vi "6（接收方）.vi"() -> ()   [LabVIEW 2017]
panel:
  in  "停止":bool
  out "波形图表":dbl(graph)
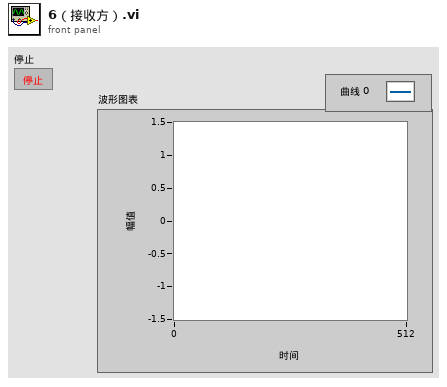
[diagram p1: front panel]
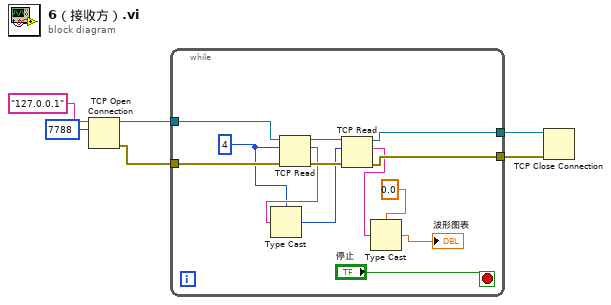
[diagram p0: block diagram]
diagram:
  n1 = TCP Open Connection(address="127.0.0.1" ("地址"), remote port or service name=u16 7788 ("远程端口或服务名称")) -> (connection ID=w6:refnum<k5>, error out=w5:errorcluster)  [unwired: 3 in]
  n2 = while {
    tunnel: w6 -> [w19]
    tunnel: w5 -> [w18]
    tunnel: [w12] -> w4
    tunnel: [w11] -> w3
    stop <- "停止" stop-if-true
    w14 = 4 ("读取的字节")
    n3 = TCP Read(connection ID=w19, bytes to read=w14, error in (no error)=w18) -> (connection ID out=w17:refnum<k5>, data out=w15:string, error out=w16:errorcluster)  [unwired: 2 in]
    n4 = Type Cast(type=w14, x=w15) -> (*(type *) &x=w13:i32)
    n5 = TCP Read(connection ID=w17, bytes to read=w13, error in (no error)=w16) -> (connection ID out=w12:refnum<k5>, data out=w10:string, error out=w11:errorcluster)  [unwired: 2 in]
    n6 = Type Cast(type=0.0, x=w10) -> (*(type *) &x=→"波形图表":dbl)
  }
  n7 = TCP Close Connection(connection ID=w4, error in (no error)=w3) -> ()  [unwired: 1 in, 2 out]
